vi "Initiate.vi"(8 "error in (no error)":errorcluster, 11 "VISA resource name":refnum<visa-resource-name>) -> (0 "error out":errorcluster, 3 "VISA resource name out":refnum<visa-resource-name>)   [LabVIEW 2009, in "Agilent 8000 Series.lvlib"]
doc: "Initiates a waveform acquisition. After you call this VI, the instrument leaves the Idle state and waits for a trigger.\n\n<B>Note:</B> Use this VI only with other low-level VIs. The high-level VIs automatically incorporate this functionality. This VI does not check the instrument status."
uses:
  Agilent 8000 Series.lvlib
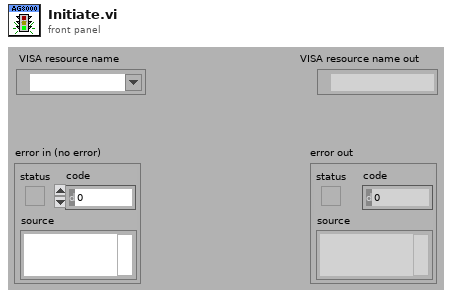
[diagram p1: front panel]
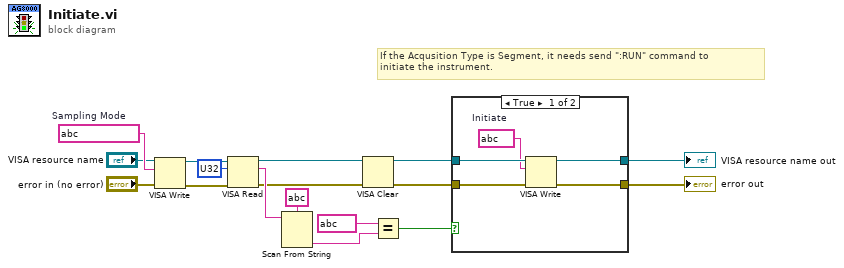
[diagram p0: block diagram]
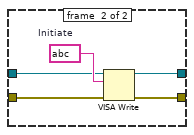
[diagram p2: hidden frame]
diagram:
  w12 = string ?  # Sampling Mode
  # "If the Acqusition Type is Segment, it needs send \":RUN\" command to\ninitiate the instrument."
  n1 = VISA Write(VISA resource name="VISA resource name", write buffer=w12, error in (no error)="error in (no error)") -> (VISA resource name out=w11:refnum<visa-resource-name>, error out=w10:errorcluster)  [unwired: 1 out]
  n2 = VISA Read(VISA resource name=w11, byte count=u32 ?, error in (no error)=w10) -> (VISA resource name out=w6:refnum<visa-resource-name>, read buffer=w15:string, error out=w5:errorcluster)  [unwired: 1 out]
  n3 = Scan From String(format string=string ?, input string=w15) -> (output 1=w1:string)  [unwired: 3 in, 3 out]
  n4 = VISA Clear(VISA resource name=w6, error in (no error)=w5) -> (VISA resource name out=w4:refnum<visa-resource-name>, error out=w3:errorcluster)
  n5 = Equal?(x=string ?, y=w1) -> (x = y?=w7:bool)
  n6 = case shown="True" w7 {
    tunnel: [w21 w26] -> w17
    tunnel: [w19 w25] -> w16
    tunnel: w4 -> [w22 w24]
    tunnel: w3 -> [w20 w23]
    frame #0 {
      w18 = string ?  # Initiate
      n7 = VISA Write(VISA resource name=w22, write buffer=w18, error in (no error)=w20) -> (VISA resource name out=w21:refnum<visa-resource-name>, error out=w19:errorcluster)  [unwired: 1 out]
    }
    frame #1 {
      w27 = string ?  # Initiate
      n8 = VISA Write(VISA resource name=w24, write buffer=w27, error in (no error)=w23) -> (VISA resource name out=w26:refnum<visa-resource-name>, error out=w25:errorcluster)  [unwired: 1 out]
    }
  }
  "error out" <- w16
  "VISA resource name out" <- w17
